vi "Get 1-Rayleigh Parameters (SubVI).vi"(6 "Flow Peak Amp.":dbl, 8 "T_Flow Start (s)":dbl, 9 "T_Flow Peak (s)":dbl, 10 "T_Ejection period (s)":dbl, 11 "Pressure (mmHg)":waveform(dbl)) -> (3 "Optimised Parameter":dbl[](array[numeric]))   [LabVIEW 2017]
uses:
  72fe1329-4430-4fd7-86c8-dfab2f7b2d2e.vi
  5c84d562-1cd3-438d-9587-7d7d9e0fcbf7.vi
panel:
  out "sorted 2D array":dbl[][](array[numeric])
  out "x-1":i32
  out "sorted array of params":dbl[][](array[numeric])
  out "Error Checks":dbl[][](array[numeric])
  out "Parameters":dbl[][](array[numeric])
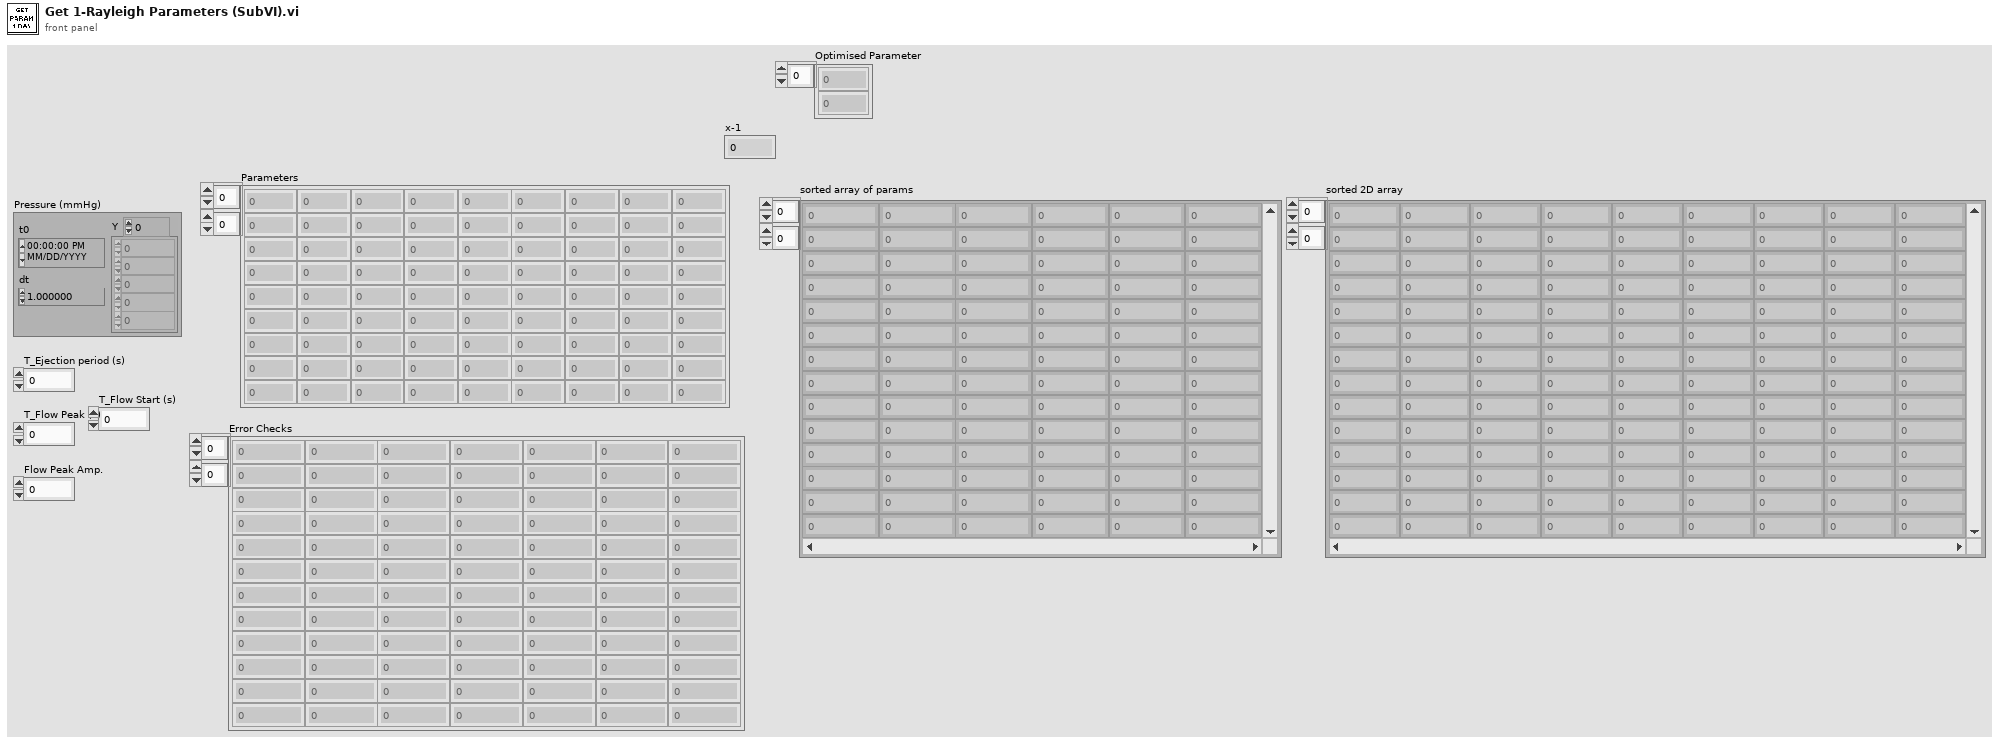
[diagram p1: front panel]
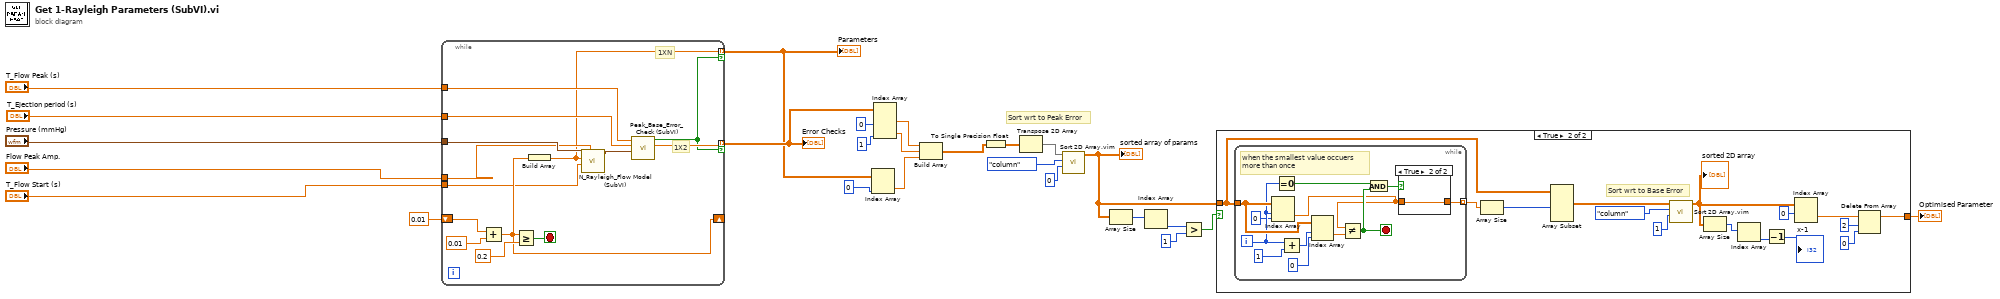
[diagram p0: block diagram]
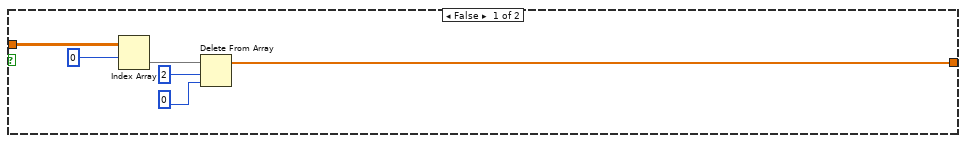
[diagram p2: hidden frame]
diagram:
  # "Sort wrt to Peak Error"
  n1 = while {
    tunnel: "Pressure (mmHg)" -> [w30]
    tunnel: "Flow Peak Amp." -> [w29]
    shift-right: [w31] -> _
    shift-left: 0.01 ("start") -> [w37]
    tunnel: "T_Ejection period (s)" -> [w35]
    tunnel: "T_Flow Peak (s)" -> [w34]
    tunnel: [w28] -> w12 mode=indexing if=w32
    tunnel: [w33] -> w16 mode=indexing if=w32
    tunnel: "T_Flow Start (s)" -> [w27]
    stop <- w36 stop-if-true
    # "1X2"
    # "1XN"
    n2 = Add(x=w37, y=0.01 ("start")) -> (x+y=w31:dbl)
    n3 = Greater Or Equal?(x=w31, y=0.2 ("start")) -> (x >= y?=w36:bool)
    n4 = Build Array(w31) -> (w28:dbl[])
    n5 = call "N_Rayleigh_Flow Model (SubVI).vi"("PSQ (ml/s)"=w29, "T_Flow Start"=w27, "Parameters (1XN)"=w28, "Pressure (mmHg)"=w30) -> ("n-Rayleigh Model Flow"=w26:waveform(dbl))  [unwired: 4 in, 1 out]
    n6 = call "Peak_Base_Error_Check (SubVI).vi"("Model Flow"=w26, "T_Ejection Period (s)"=w35, "T_Flow Peak (s)"=w34) -> ("Error"=w33:dbl[], "Logic"=w32:bool)  [unwired: 5 in, 2 out]
  }
  "Parameters" <- w12
  "Error Checks" <- w16
  n7 = Index Array(array=w12, index (col)=0 ("disabled index (col)")) -> (element=w13:dbl[])  [unwired: 1 in]
  n8 = Index Array(array=w16, index (col) #1=0 ("disabled index (col)"), index (col) #2=1 ("index (col)")) -> (element #1=w15:dbl[], element #2=w14:dbl[])  [unwired: 2 in]
  n9 = Build Array(w15, w14, w13) -> (w3:dbl[][])
  n10 = To Single Precision Float(number=w3) -> (single precision float=w4:sgl[][])
  n11 = Transpose 2D Array(2D array=w4) -> (transposed array=w11:sgl[][])
  n12 = call "Sort 2D Array.vim"("index"=0, "dimension to index (column)"=enum16{"column", "row"}."column", "2D array"=w11) -> ("sorted 2D array"=w5:sgl[][])  [unwired: 7 in, 1 out]
  "sorted array of params" <- w5
  n13 = Array Size(array=w5) -> (size(s)=w9:i32[])
  n14 = Index Array(array=w9) -> (element=w8:i32)  [unwired: 1 in]
  n15 = Greater?(x=w8, y=1) -> (0:w7:bool)
  n16 = case shown="True" w7 {
    tunnel: w5 -> [w45 w49]
    tunnel: [w40 w48] -> w6
    frame False {
      n17 = Index Array(array=w45, index (row)=0) -> (element=w43:sgl[])  [unwired: 1 in]
      n18 = Delete From Array(array=w43, length=2, index=0) -> (array with subset deleted=w40:sgl[])  [unwired: 1 out]
    }
    frame True {
      # "Sort wrt to Base Error"
      n19 = while {
        tunnel: w49 -> [w70]
        tunnel: [w67] -> w50 mode=indexing
        i -> [w69]
        stop <- w63 stop-if-true
        # "when the smallest value occuers \nmore than once"
        n20 = Index Array(array=w70, index (row)=w69, index (col)=0 ("disabled index (col)")) -> (element=w62:sgl)
        n21 = Equal To 0?(x=w69) -> (x = 0?=w68:bool)
        n22 = Add(x=w69, y=1) -> (x+y=w71:i32)
        n23 = Index Array(array=w70, index (row)=w71, index (col)=0 ("disabled index (col)")) -> (element=w61:sgl)
        n24 = Not Equal?(x=w62, y=w61) -> (x != y?=w63:bool)
        n25 = And(x=w68, y=w63) -> (x .and. y?=w64:bool)
        n26 = case shown="True" w64 {
          tunnel: w62 -> [w73 w74]
          tunnel: [w73 w74] -> w67
          frame False {
          }
          frame True {
          }
        }
      }
      n27 = Array Size(array=w50) -> (size(s)=w47:i32)
      n28 = Array Subset(array=w49, length (row)=w47) -> (w55:sgl[][])  [unwired: 3 in]
      n29 = call "Sort 2D Array.vim"("index"=1, "dimension to index (column)"=enum16{"column", "row"}."column", "2D array"=w55) -> ("sorted 2D array"=w56:sgl[][])  [unwired: 7 in, 1 out]
      "sorted 2D array" <- w56
      n30 = Array Size(array=w56) -> (size(s)=w57:i32[])
      n31 = Index Array(array=w57) -> (element=w58:i32)  [unwired: 1 in]
      n32 = Decrement(x=w58) -> (x-1=→"x-1":i32)
      n33 = Index Array(array=w56, index (row)=0) -> (element=w60:sgl[])  [unwired: 1 in]
      n34 = Delete From Array(array=w60, length=2, index=0) -> (array with subset deleted=w48:sgl[])  [unwired: 1 out]
    }
  }
  "Optimised Parameter" <- w6
